vi "test1.vi"() -> ()   [LabVIEW 2016]
panel:
  out "数值 3":dbl
  in  "数值 2":dbl
  in  "数值":dbl
  # "+"
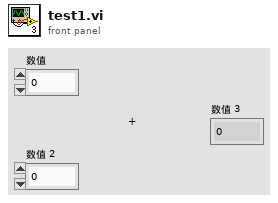
[diagram p1: front panel]
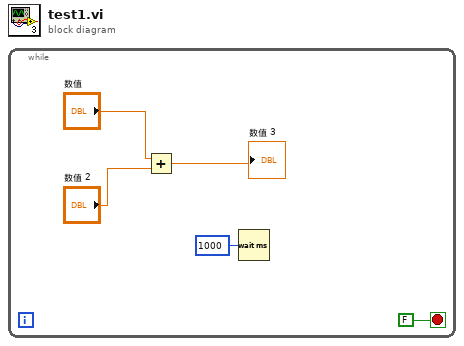
[diagram p0: block diagram]
diagram:
  n1 = while {
    stop <- FALSE stop-if-true
    n2 = Add(x="数值", y="数值 2") -> (x+y=→"数值 3":dbl)
    n3 = Wait (ms)(milliseconds to wait=u32 1000 ("等待时间（毫秒）")) -> ()  [unwired: 1 out]
  }
